vi "Low-Level HTTP Request AWS v4.vi"(4 "Object Key":string, 6 "Bucket":string, 7 "Request Options":T1, 8 "error in (no error)":errorcluster, 9 "Region":string="us-east-1", 10 "AWS Service":string="s3", 11 "HTTP-Verb":string(combo)="GET") -> (0 "error out":errorcluster, 1 "response body":string, 2 "response headers":string, 3 "Call Result":T2)   [LabVIEW 2015, in "LV Interface for Amazon S3.lvlib"]
doc: "This core implementation of AWS v4 HTTP requests may be used to implement special requests or API calls not present in this toolkit."
uses:
  LV Interface for Amazon S3.lvlib
  Typedefs/AMZ_S3_Call Results.ctl
  Typedefs/AMZ_S3_API_Request Options.ctl
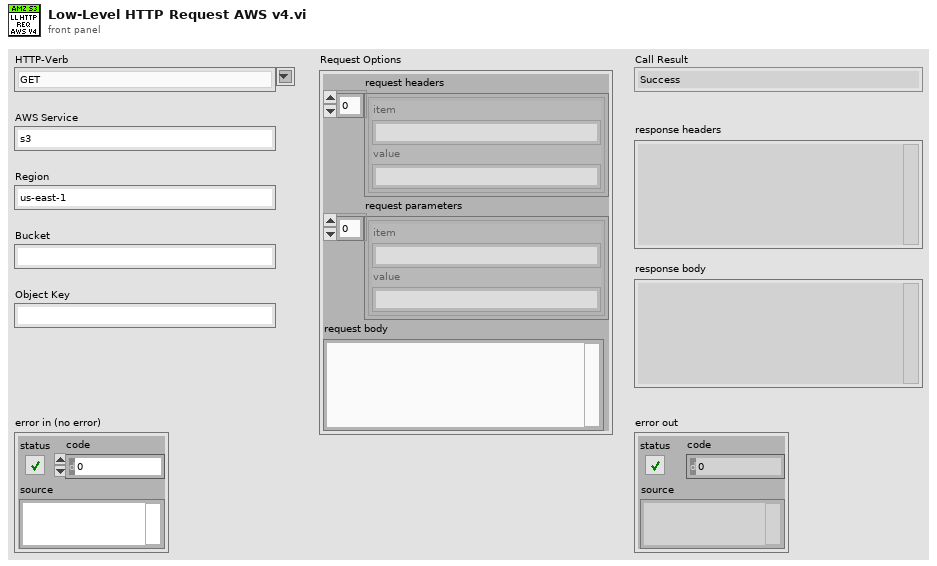
[diagram p1: front panel]
types:
  T1 = typedef "LV Interface for Amazon S3.lvlib/AMZ_S3_API_Request Options.ctl" = cluster{"request headers":cluster{"item":string, "value":string}[], "request parameters":cluster{"item":string, "value":string}[], "request body":string}
  T2 = typedef "LV Interface for Amazon S3.lvlib/AMZ_S3_Call Results.ctl" = enum16{"Success", "UndefinedError", "AccessDenied", "AccountProblem", "AmbiguousGrantByEmailAddress", "BadDigest", "BucketAlreadyExists", "BucketAlreadyOwnedByYou", "BucketNotEmpty", "CredentialsNotSupported", "CrossLocationLoggingProhibited", "EntityTooSmall", "EntityTooLarge", "ExpiredToken", "IllegalVersioningConfigurationException", "IncompleteBody", "IncorrectNumberOfFilesInPostRequest", "InlineDataTooLarge", "InternalError", "InvalidAccessKeyId", "InvalidAddressingHeader", "InvalidArgument", "InvalidBucketName", "InvalidDigest", "InvalidLocationConstraint", "InvalidPart", "InvalidPartOrder", "InvalidPayer", "InvalidPolicyDocument", "InvalidRange", "InvalidSecurity", "InvalidSOAPRequest", "InvalidStorageClass", "InvalidTargetBucketForLogging", "InvalidToken", "InvalidURI", "KeyTooLong", "MalformedACLError", "MalformedPOSTRequest", "MalformedXML", "MaxMessageLengthExceeded", "MaxPostPreDataLengthExceededError", "MetadataTooLarge", "MethodNotAllowed", "MissingAttachment", "MissingContentLength", "MissingRequestBodyError", "MissingSecurityElement", "MissingSecurityHeader", "NoLoggingStatusForKey", "NoSuchBucket", "NoSuchKey", "NoSuchUpload", "NoSuchVersion", "NotImplemented", "NotSignedUp", "OperationAborted", "PermanentRedirect", "PreconditionFailed", "Redirect", "RequestIsNotMultiPartContent", "RequestTimeout", "RequestTimeTooSkewed", "RequestTorrentOfBucketError", "SignatureDoesNotMatch", "SlowDown", "TemporaryRedirect", "TokenRefreshRequired", "TooManyBuckets", "UnexpectedContent", "UnresolvableGrantByEmailAddress", "UserKeyMustBeSpecified", "LabVIEWError"}
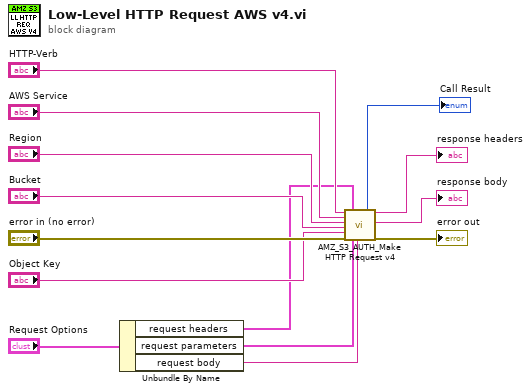
[diagram p0: block diagram]
diagram:
  n1 = Unbundle By Name("Request Options") -> ("request headers"=w3:cluster{"item":string, "value":string}[], "request parameters"=w2:cluster{"item":string, "value":string}[], "request body"=w1:string)
  n2 = call "AMZ_S3_AUTH_Make HTTP Request v4.vi"("HTTP-Verb"="HTTP-Verb", "AWS Service"="AWS Service", "Region"="Region", "Bucket"="Bucket", "Object Key"="Object Key", "error in"="error in (no error)", "request headers"=w3, "request parameters"=w2, "request body"=w1) -> ("Call Result"=→"Call Result":T2, "response headers"=→"response headers":string, "response body"=→"response body":string, "error out"=→"error out":errorcluster)  [unwired: 7 in]
